vi "Air.vi"(1 "temperature adjustment":dbl[unit]) -> (0 "new air temperature":dbl[unit]=273.15)   [LabVIEW 2023]
doc: "This VI represents the simulated air temperature. Various other VIs will call this to simulate heating or cooling the air in the testing chamber. Passing NaN will reset the chamber to a balmy 30 degrees Celsius."
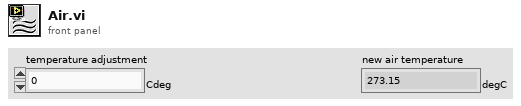
[diagram p1: front panel]
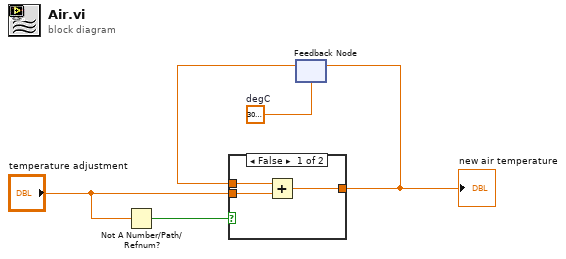
[diagram p0: block diagram]
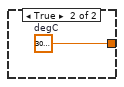
[diagram p2: hidden frame]
diagram:
  w2 = dbl[unit] 303.15  # degC
  n1 = Not A Number/Path/Refnum?(number/path/refnum="temperature adjustment") -> (NaN/Path/Refnum?=w3:bool)
  n2 = feedback #1(w2) -> (w5:dbl[unit])
  n3 = case shown="False" w3 {
    tunnel: w5 -> [w8 _]
    tunnel: [w7 w9] -> w1
    tunnel: "temperature adjustment" -> [w6 _]
    frame False {
      n4 = Add(x=w8, y=w6) -> (x+y=w7:dbl[unit])
    }
    frame True {
      w9 = dbl[unit] 303.15  # degC
    }
  }
  "new air temperature" <- w1
  n5 = feedback-in #1(w1) -> ()
